vi "Process.vi"(8 "error in":errorcluster, 11 "Instrument.Example":refnum<class "Instrument.OxfordVRM.lvclass">) -> (0 "error out":errorcluster, 3 "Instrument.Example out":refnum<class "Instrument.OxfordVRM.lvclass">)   [LabVIEW 2016, in "Instrument.OxfordVRM.lvclass"]
doc: "---------------------------------------------------------------\nJKI State Machine Objects™\nhttp://jki.net/state-machine-objects/\nCopyright (C) 2005-2015, JKI <info@jki.net>\nALL RIGHTS RESERVED"
uses:
  Instrument.OxfordVRM.lvclass
  <vilib>/JKI/JKI SMO/SMO/SMO.lvclass
  <vilib>/JKI/JKI SMO/SMO/Typedefs/Parent Call--Enum.ctl
  <userlib>/LevyLab/Levylab Instruments/Instrument Types/Cryostat/Instrument.Cryostat.lvclass
  C:/Program Files (x86)/National Instruments/LabVIEW 2016/user.lib/LevyLab/Levylab Instruments/Instrument Types/Cryostat/Instrument.Cryostat.lvclass
  C:/Program Files (x86)/National Instruments/LabVIEW 2016/user.lib/LevyLab/Levylab Instruments/SMOs/Instrument/Instrument.lvclass
  C:/Program Files (x86)/National Instruments/LabVIEW 2016/vi.lib/JKI/JKI SMO/SMO/SMO.lvclass
  <userlib>/LevyLab/Levylab Instruments/Instrument Types/Cryostat/Typedefs/VRM Magnet Axis--Enum.ctl
panel:
  out "State":string
  out "timer":u32
  # "For instructions on how to use the JKI State Machine Objects, examples and video tutorials, visit:\nhttp://jki.net/state-machine-objects/\n\nJKI State Machine Objects™\nhttp://jki.net/state-machine-objects/\nCopyright (C) 2005-2015, JKI <info@jki.net>\nALL RIGHTS RESERVED"
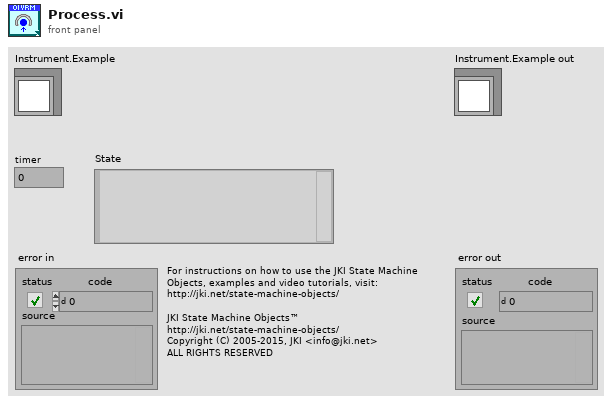
[diagram p1: front panel]
types:
  T1 = typedef "SMO.lvclass/Parent Call--Enum.ctl" = enum16{"Allows parent to run", "Does not request parent to run"}
  T2 = enum32{"invalid app kind", "Development System", "Run Time System", "Student Edition", "Embedded LabVIEW", "Evaluation", "Custom"}
  T3 = enum32{"Invalid", "Standard", "Closed", "Hidden", "Minimized", "Maximized"}
  T4 = enum32{"Bad", "Idle", "Run top level", "Running"}
  T5 = typedef "Instrument.OxfordVRM.lvclass/VRM Magnet Axis--Enum.ctl" = enum16{"Z", "X", "Y", "ALL"}
  T6 = cluster{"Core":cluster{"Current VI Reference":refnum<vi>, "Close Panel on Exit?":bool, "error":errorcluster}, "Self Reference":refnum<class "Instrument.OxfordVRM.lvclass">, "Field (T)":dbl, "Field Rate (T/min)":dbl, "Axis":T5, "Running Step":i32, "sequence":string[]}
  T7 = cluster{"Current VI Reference":refnum<vi>, "Close Panel on Exit?":bool, "error":errorcluster}
  T8 = typedef "SMO.lvclass/Protected Events.ctl" = cluster{"StopProcesses":refnum<user-event>, "AbortProcesses":refnum<user-event>, "Config Changed":refnum<user-event>, "Dependency":refnum<user-event>}
  T9 = typedef "Instrument.OxfordVRM.lvclass/PrivateEvents--Cluster.ctl" = cluster{"SequenceSetMagnetField":refnum<user-event>, "AbortSequence":refnum<user-event>}
  T10 = cluster{"Holding":bool, "Ramp to Setpoint":bool, "Ramp to Zero":bool, "Clamp":bool}
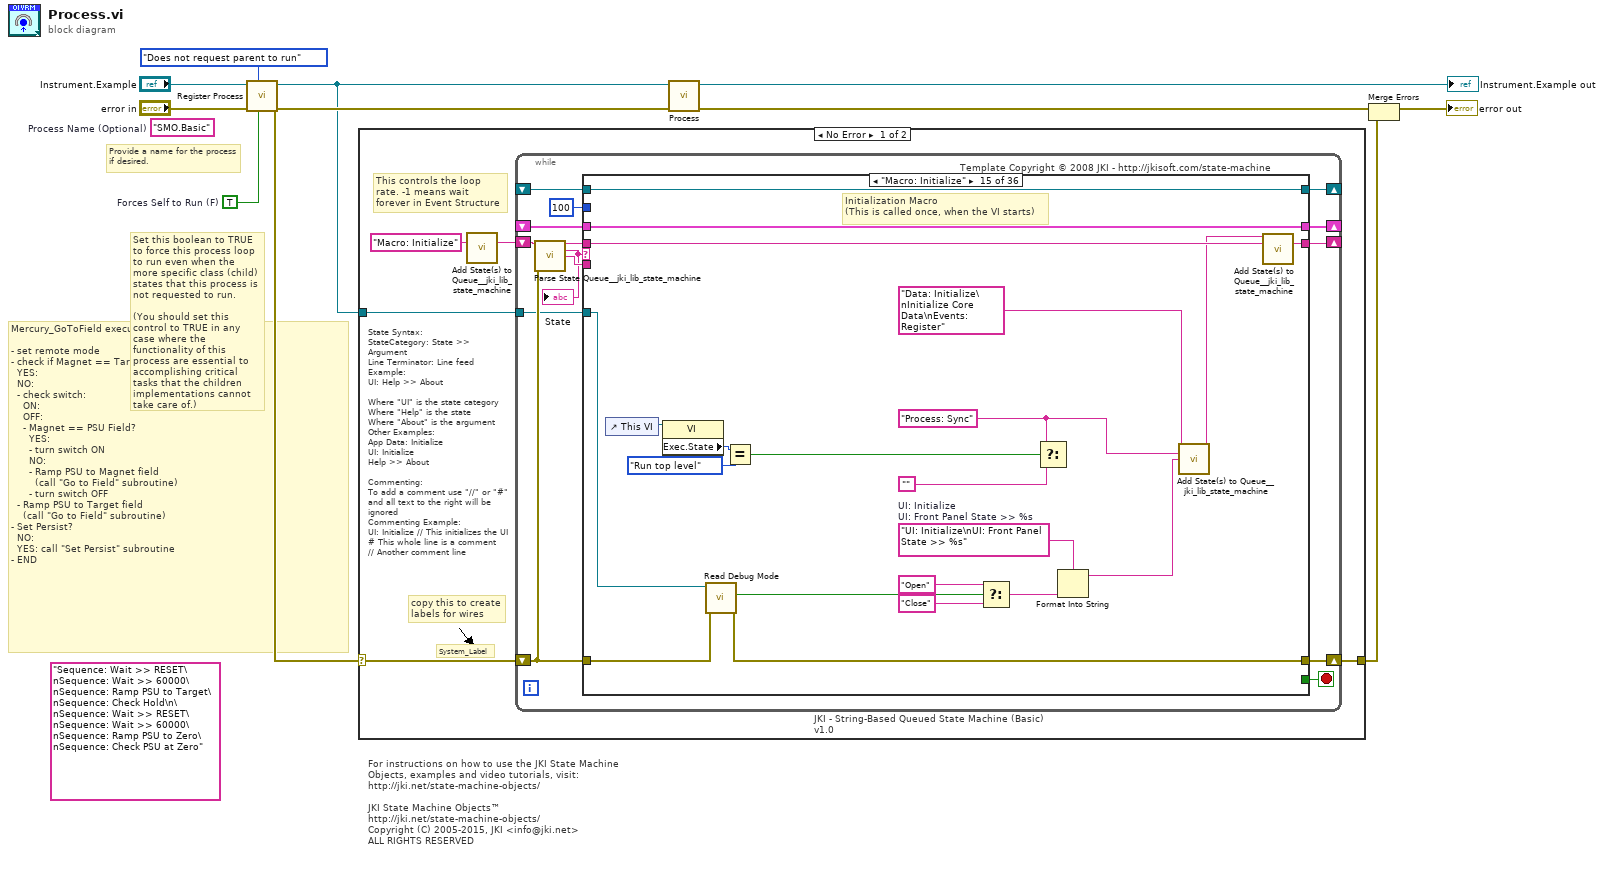
[diagram p0: block diagram]
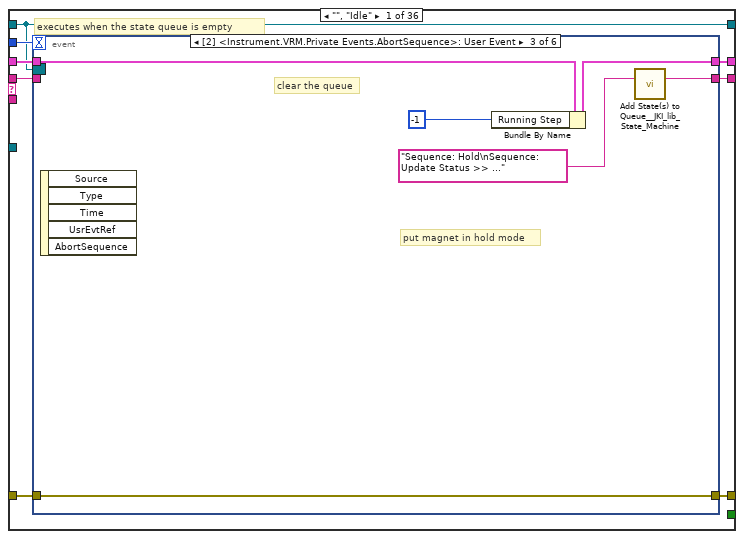
[diagram p2: hidden frame]
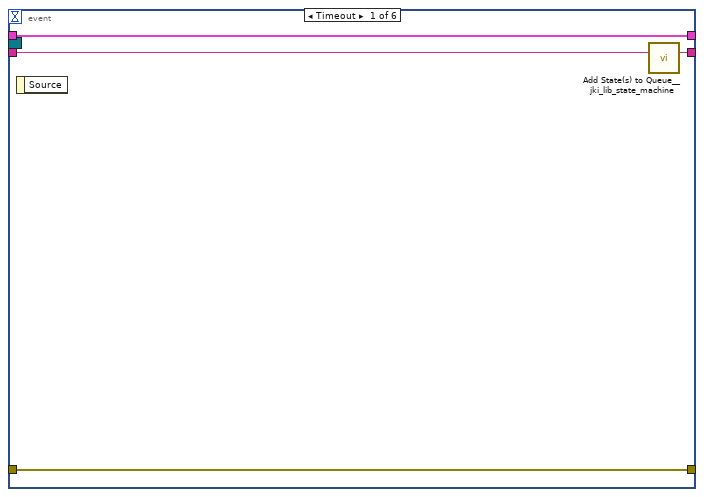
[diagram p3: hidden frame]
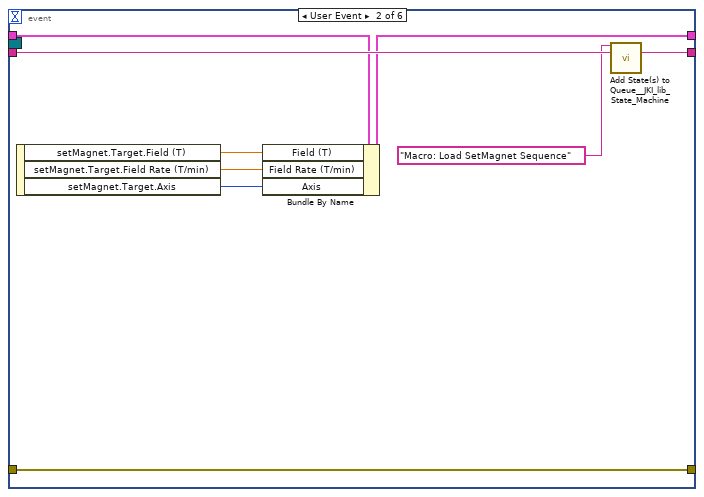
[diagram p4: hidden frame]
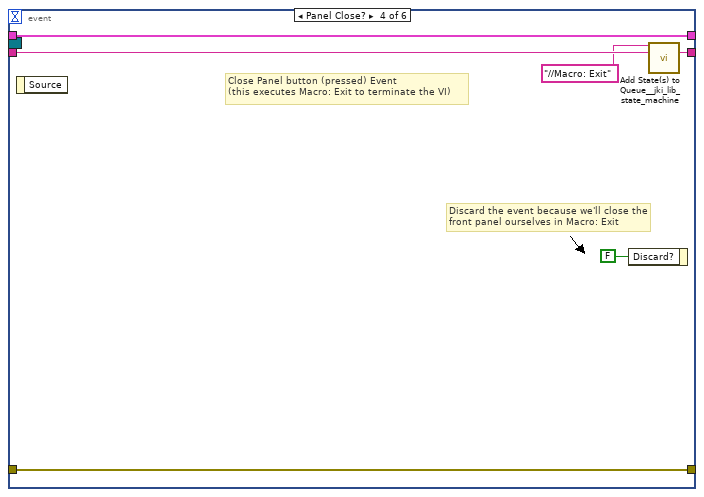
[diagram p5: hidden frame]
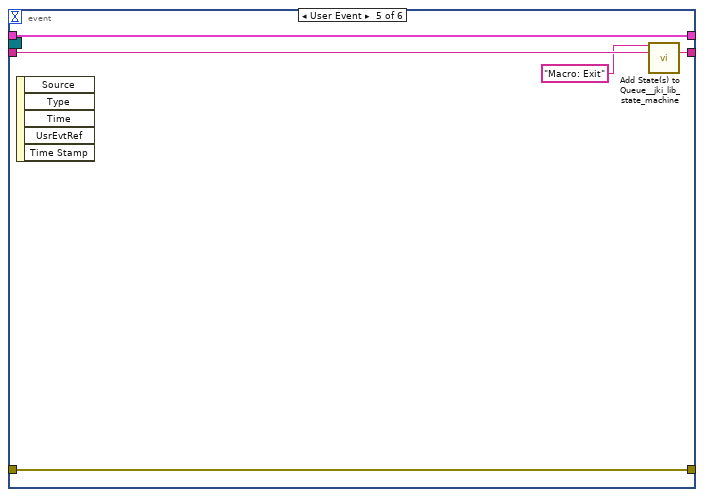
[diagram p6: hidden frame]
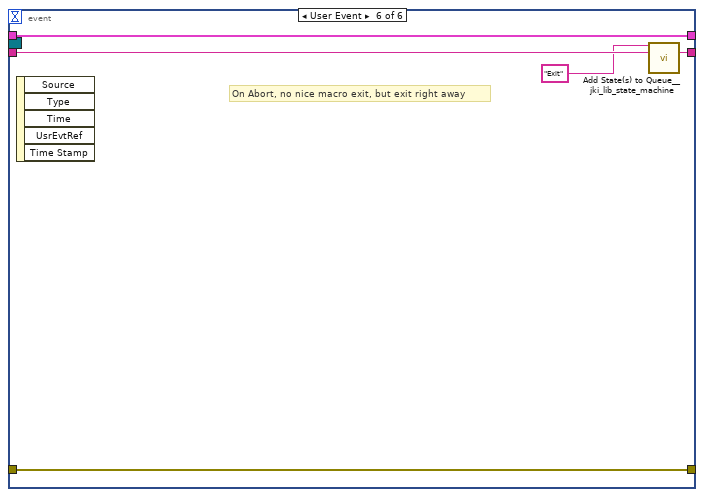
[diagram p7: hidden frame]
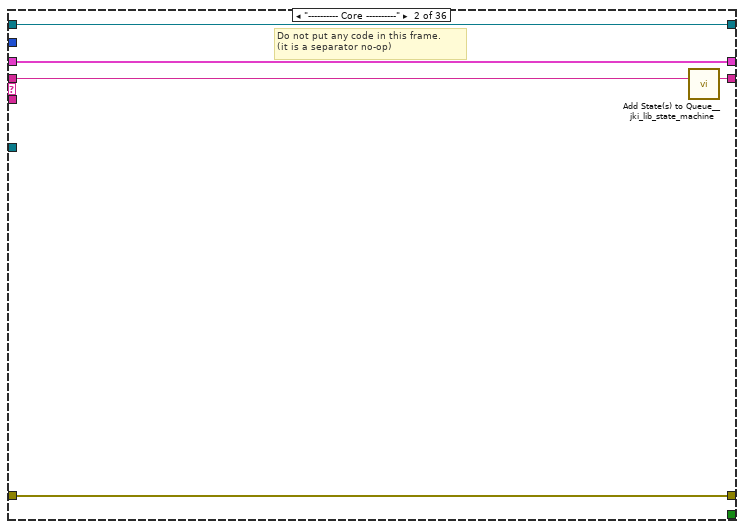
[diagram p8: hidden frame]
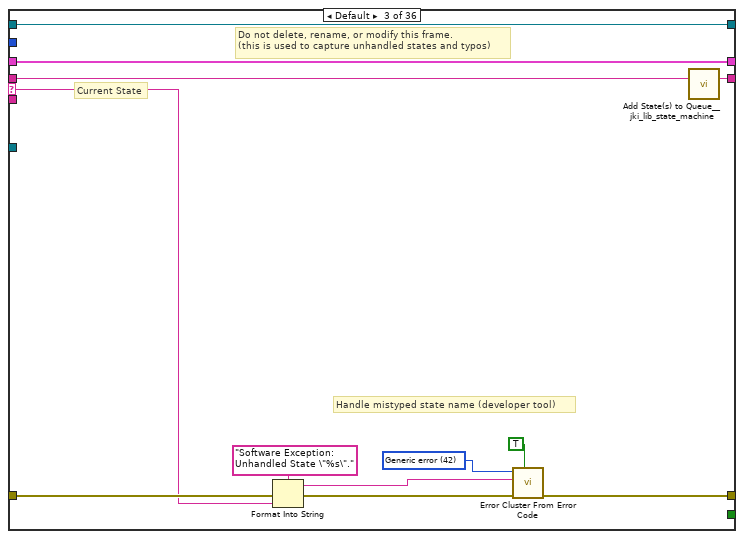
[diagram p9: hidden frame]
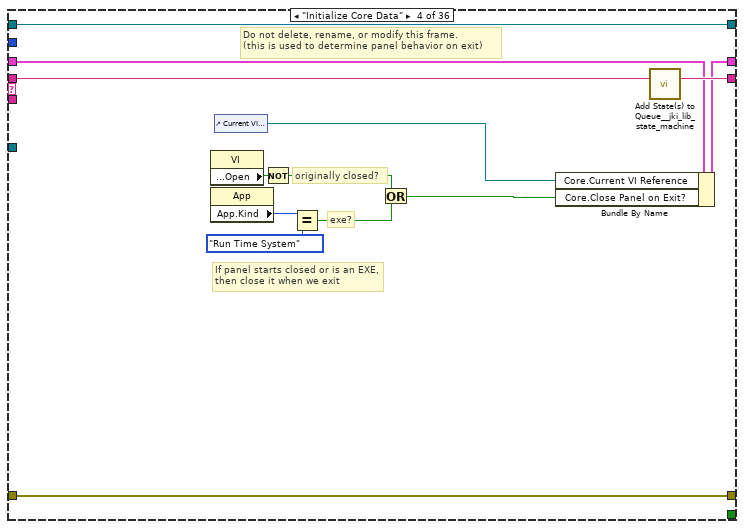
[diagram p10: hidden frame]
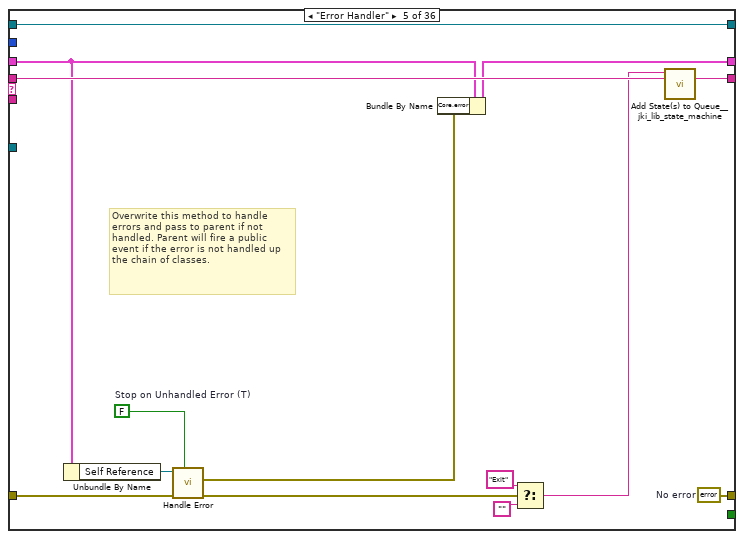
[diagram p11: hidden frame]
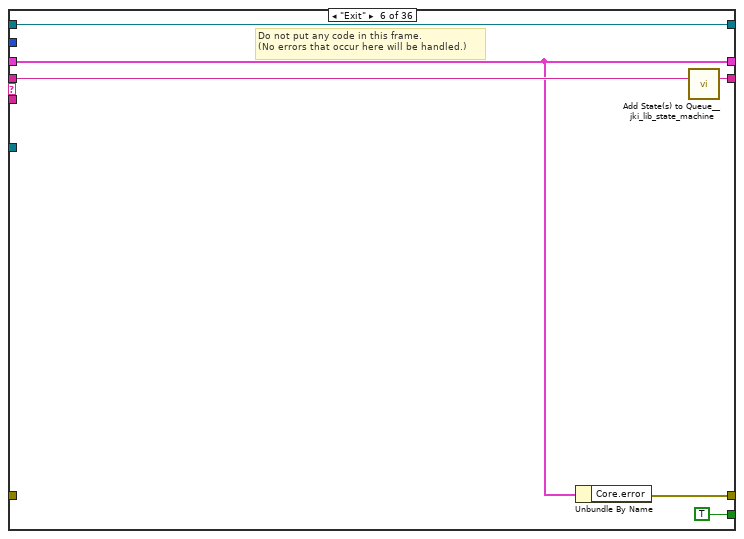
[diagram p12: hidden frame]
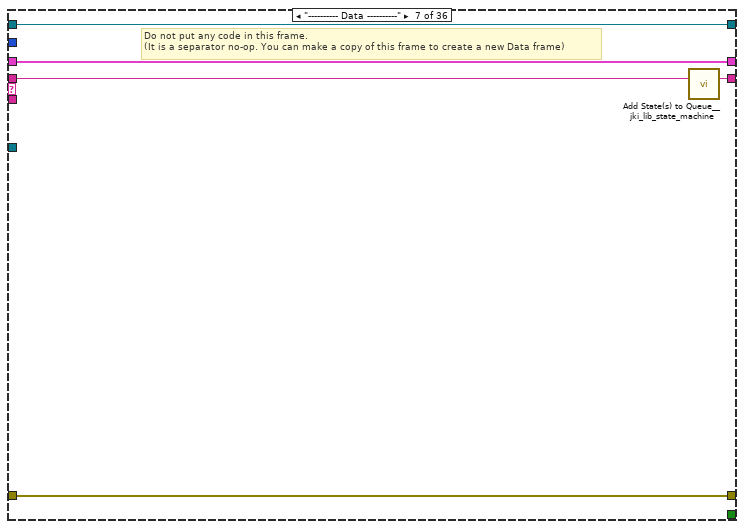
[diagram p13: hidden frame]
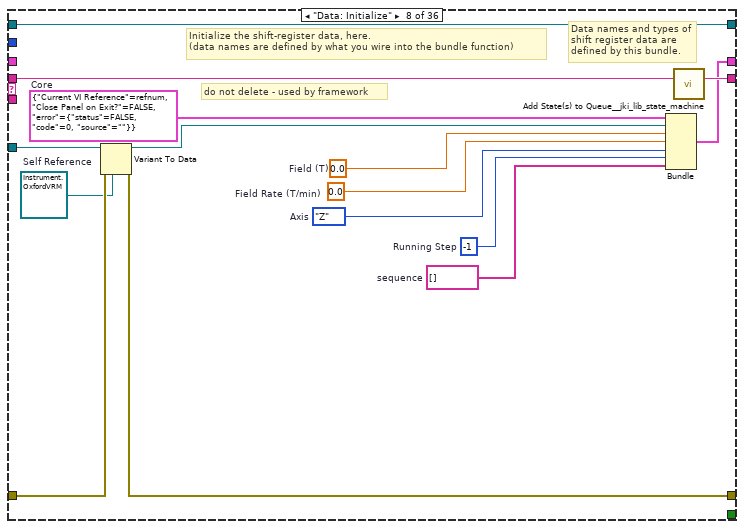
[diagram p14: hidden frame]
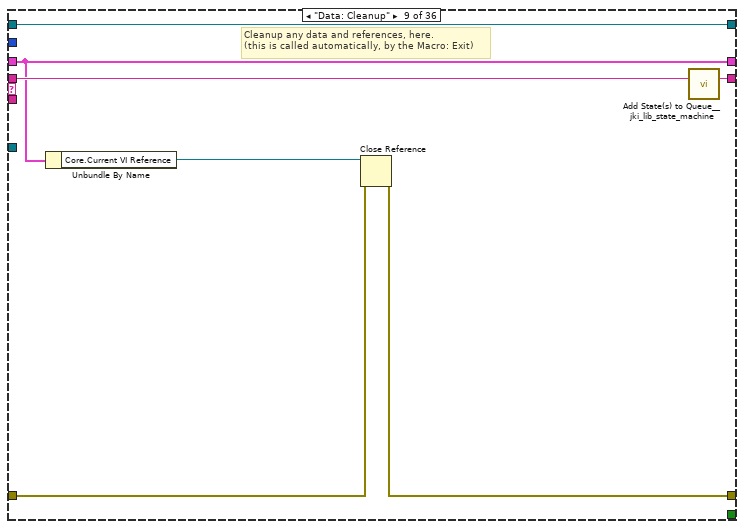
[diagram p15: hidden frame]
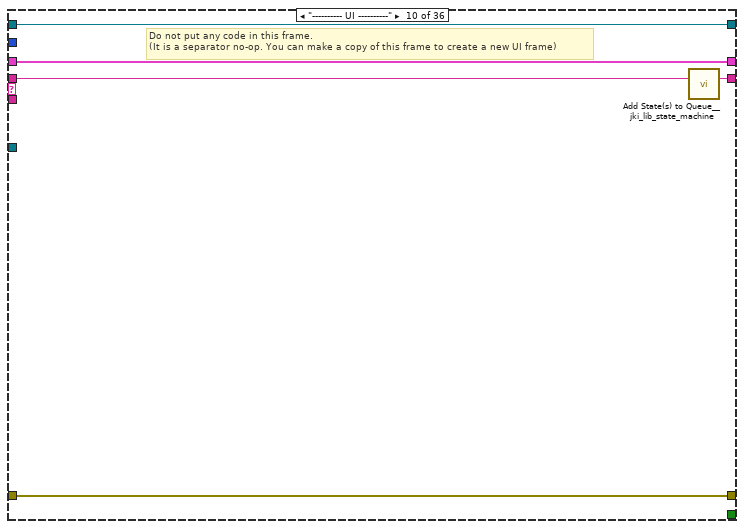
[diagram p16: hidden frame]
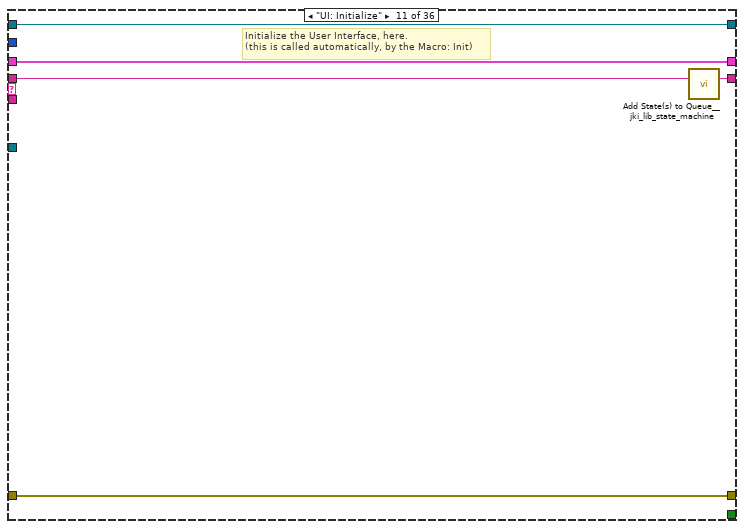
[diagram p17: hidden frame]
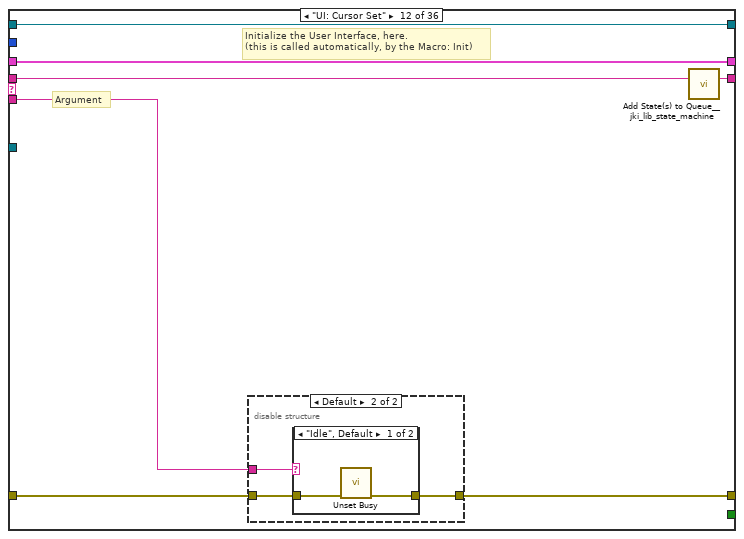
[diagram p18: hidden frame]
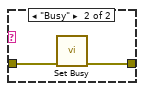
[diagram p20: hidden frame]
diagram:
  (unwired) "Sequence: Wait >> RESET\nSequence: Wait >> 60000\nSequence: Ramp PSU to Target\nSequence: Check Hold\n\nSequence: Wait >> RESET\nSequence: Wait >> 60000\nSequence: Ramp PSU to Zero\nSequence: Check PSU at Zero" ("State(s) in Front (\"\")")
  w1 = TRUE  # Forces Self to Run (F)
  (unwired) "SMO.Basic"  # Process Name (Optional)
  # "Mercury_GoToField executes the following states:\n\n- set remote mode\n- check if Magnet == Target.\n  YES:\n  NO:\n  - check switch:\n    ON:\n    OFF:\n    - Magnet == PSU Field?\n      YES:\n      - turn switch ON\n      NO:\n      - Ramp PSU to Magnet field\n        (call \"Go to Field\" subroutine)\n      - turn switch OFF\n  - Ramp PSU to Target field\n    (call \"Go to Field\" subroutine)\n- Set Persist?\n  NO:\n  YES: call \"Set Persist\" subroutine\n- END"
  # "Provide a name for the process\nif desired."
  # "Set this boolean to TRUE to force this process loop to run even when the more specific class (child) states that this process is not requested to run.\n\n(You should set this control to TRUE in any case where the functionality of this process are essential to accomplishing critical tasks that the children implementations cannot take care of.)"
  # "For instructions on how to use the JKI State Machine Objects, examples and video tutorials, visit:\nhttp://jki.net/state-machine-objects/\n\nJKI State Machine Objects™\nhttp://jki.net/state-machine-objects/\nCopyright (C) 2005-2015, JKI <info@jki.net>\nALL RIGHTS RESERVED"
  n1 = call <vilib>:"Register Process.vi"("Forces Self to Run (F)"=w1, "Parent Call"=Parent_Call--Enum."Does not request parent to run", "error in (no error)"="error in", "SMO"="Instrument.Example") -> ("error out"=w7:errorcluster, "SMO out"=w6:refnum<class "Instrument.OxfordVRM.lvclass">)  [unwired: 6 in]
  n2 = case shown="No Error" w7 {
    selector: w7 -> [w12 w596]
    tunnel: w6 -> [w13 _]
    tunnel: [w11 w596] -> w3
    frame No Error {
      # "State Syntax:\nStateCategory: State >> Argument\nLine Terminator: Line feed\nExample:\nUI: Help >> About\n\nWhere \"UI\" is the state category\nWhere \"Help\" is the state\nWhere \"About\" is the argument\nOther Examples:\nApp Data: Initialize\nUI: Initialize\nHelp >> About\n\nCommenting:\nTo add a comment use \"//\" or \"#\" and all text to the right will be ignored\nCommenting Example:\nUI: Initialize // This initializes the UI\n# This whole line is a comment\n// Another comment line"
      # "copy this to create labels for wires"
      # "This controls the loop rate. -1 means wait forever in Event Structure"
      # "System_Label"
      n3 = call <vilib>:"Add State(s) to Queue__jki_lib_state_machine.vi"("State(s) in (\"\")"="Macro: Initialize") -> ("States Out"=w15:string)  [unwired: 14 in]
      n4 = while "JKI - String-Based Queued State Machine (Basic) v1.0" {
        shift-right: [w23] -> _
        shift-left: _ -> [w22]
        shift-right: [w26] -> w11
        shift-left: w12 -> [w20]
        shift-right: [w25] -> _
        shift-left: w15 -> [w27]
        tunnel: w13 -> [w19]
        shift-right: [w18] -> _
        shift-left: _ -> [w17]
        stop <- w24 stop-if-true
        # "Template Copyright © 2008 JKI - http://jkisoft.com/state-machine"
        n5 = call <vilib>:"Parse State Queue__jki_lib_state_machine.vi"("State Queue"=w27, "Error In (no error)"=w20) -> ("Remaining States"=w29:string, "Current State"=w16:string, "Arguments"=w28:string)  [unwired: 11 in]
        "State" <- w16
        n6 = case shown="\"Macro: Initialize\"" w16 {
          selector: w16 -> [_ _ w79 _ _ _ _ _ _ _ _ _ _ _ _ _ _ _ _ _ _ _ _ _ _ _ w360 w385 w410 w441 w475 w494 w515 w536 w555 w586]
          tunnel: w29 -> [w37 w77 w83 w102 w116 w122 w127 w142 w149 w154 w159 w166 w182 w214 w235 w249 w266 _ w293 w304 w309 w322 w328 w337 w344 w354 w369 w398 w426 w458 w483 w504 w525 w546 w567 w595]
          tunnel: w28 -> [_ _ _ _ _ _ _ _ _ _ _ w160 w176 _ _ _ _ _ _ _ _ _ _ _ _ w346 _ w386 _ _ _ _ _ _ _ _]
          tunnel: w22 -> [w35 w74 w81 w93 w110 w118 w124 _ w144 w151 w157 w164 w178 w211 w232 w240 w254 w275 w290 w301 w306 w320 w326 w331 w340 w345 w366 w371 w419 w454 w480 w497 w518 w539 w564 w592]
          tunnel: [w34 w75 w85 w99 w111 w117 w125 w138 w145 w152 w156 w161 w179 w212 w215 w247 w264 w271 w291 w295 w307 w315 w324 w334 w341 w348 w363 w375 w413 w450 w471 w486 w507 w528 w547 w585] -> w26
          tunnel: w20 -> [w33 w75 w84 w99 w112 _ w125 w139 w146 w152 w156 w162 w180 w212 w216 w247 w264 w272 w291 w296 w307 w316 w324 w334 w341 w349 w358 w374 w408 w439 w472 w484 w506 w527 w549 w580]
          tunnel: [w36 w76 w82 w101 w115 w121 w126 w141 w148 w153 w158 w165 w181 w213 w234 w248 w265 w281 w292 w303 w308 w321 w327 w336 w343 w353 w368 w397 w425 w457 w482 w503 w524 w545 w566 w594] -> w25
          tunnel: [_ _ _ _ _ TRUE _ _ _ _ _ _ _ _ _ _ _ _ _ _ _ _ _ _ _ _ _ _ _ _ _ _ _ _ _ _] -> w24
          tunnel: [w32 w74 w81 w100 w109 w118 w124 w140 w144 w151 w157 w164 w178 w211 w232 w240 w262 w276 w290 w301 w306 w320 w326 w330 w339 w351 w365 w395 w418 w453 w479 w496 w517 w538 w563 w591] -> w23
          tunnel: 100 ("Timeout") -> [w31 _ _ _ _ _ _ _ _ _ _ _ _ _ _ _ _ _ _ _ _ _ _ _ _ _ _ _ _ _ _ _ _ _ _ _]
          tunnel: w19 -> [_ _ _ _ _ _ _ w136 _ _ _ _ _ _ w223 _ _ _ _ _ _ _ _ _ _ _ _ _ _ _ _ _ _ _ _ _]
          tunnel: [w30 w73 w78 w90 w114 w119 w123 w134 w143 w150 w155 w163 w175 w210 w233 w241 w263 w280 w289 w302 w305 w319 w325 w335 w342 w352 w367 w396 w424 w456 w481 w502 w523 w544 w565 w593] -> w18
          tunnel: w17 -> [w30 w73 w78 w90 w114 w119 w123 w134 w143 w150 w155 w163 w175 w210 w233 w241 w263 w280 w289 w302 w305 _ w325 w335 w342 w352 w367 w396 w424 w456 w481 w502 w523 w544 w565 w593]
          frame "", "Idle" {
            # "executes when the state queue is empty"
            n7 = event shown="[2] <Instrument.VRM.Private Events.AbortSequence>: User Event" {
              selector: w30 -> [_ _ _ _ _ _]
              dyn-events: _ -> [_ _ _ _ _ _]
              timeout: w31 -> [_ _ _ _ _ _]
              tunnel: w37 -> [w41 w48 _ w62 w67 w72]
              tunnel: [w40 w49 w55 w61 w66 w71] -> w36
              tunnel: w35 -> [w38 w45 w53 w59 w64 w69]
              tunnel: [w39 w50 w56 w60 w65 w70] -> w34
              tunnel: w33 -> [w39 w50 w56 w60 w65 w70]
              tunnel: [w38 w44 w52 w59 w64 w69] -> w32
              event Timeout {
                n8 = event-data() -> ()  [unwired: 1 in, 1 out]
                n9 = call <vilib>:"Add State(s) to Queue__jki_lib_state_machine.vi"("State(s) in (\"\")"=w41) -> ("States Out"=w40:string)  [unwired: 14 in]
              }
              event User Event {
                n10 = event-data() -> ("setMagnet.Target.Field (T)"=w47:dbl, "setMagnet.Target.Field Rate (T/min)"=w46:dbl, "setMagnet.Target.Axis"=w42:T5)  [unwired: 1 in]
                n11 = Bundle By Name(cluster=w45, "Field (T)"=w47, "Field Rate (T/min)"=w46, "Axis"=w42) -> (w44:T6)
                n12 = call <vilib>:"Add State(s) to Queue__JKI_lib_State_Machine.vi"("State(s) in Front (\"\")"="Macro: Load SetMagnet Sequence" ("State(s) at Back (\"\")"), "State(s) in (\"\")"=w48) -> ("States Out"=w49:string)  [unwired: 13 in]
              }
              event User Event {
                # "put magnet in hold mode"
                # "clear the queue"
                n13 = event-data() -> ()  [unwired: 1 in, 5 out]
                n14 = Bundle By Name(cluster=w53, "Running Step"=-1) -> (w52:T6)
                n15 = call <vilib>:"Add State(s) to Queue__JKI_lib_State_Machine.vi"("State(s) in (\"\")"="Sequence: Hold\nSequence: Update Status >> ..." ("State(s) at Back (\"\")")) -> ("States Out"=w55:string)  [unwired: 14 in]
              }
              event Panel Close? {
                # "Discard the event because we'll close the front panel ourselves in Macro: Exit"
                # "Close Panel button (pressed) Event\n(this executes Macro: Exit to terminate the VI)"
                n16 = event-data() -> ()  [unwired: 1 in, 1 out]
                n17 = event-data("Discard?"=FALSE) -> ()  [unwired: 1 in, 1 out]
                n18 = call <vilib>:"Add State(s) to Queue__jki_lib_state_machine.vi"("State(s) in Front (\"\")"="//Macro: Exit", "State(s) in (\"\")"=w62) -> ("States Out"=w61:string)  [unwired: 13 in]
              }
              event User Event {
                n19 = event-data() -> ()  [unwired: 1 in, 5 out]
                n20 = call <vilib>:"Add State(s) to Queue__jki_lib_state_machine.vi"("State(s) in Front (\"\")"="Macro: Exit", "State(s) in (\"\")"=w67) -> ("States Out"=w66:string)  [unwired: 13 in]
              }
              event User Event {
                # "On Abort, no nice macro exit, but exit right away"
                n21 = event-data() -> ()  [unwired: 1 in, 5 out]
                n22 = call <vilib>:"Add State(s) to Queue__jki_lib_state_machine.vi"("State(s) in Front (\"\")"="Exit", "State(s) in (\"\")"=w72) -> ("States Out"=w71:string)  [unwired: 13 in]
              }
            }
          }
          frame "---------- Core ----------" {
            # "Do not put any code in this frame.\n(it is a separator no-op)"
            n23 = call <vilib>:"Add State(s) to Queue__jki_lib_state_machine.vi"("State(s) in (\"\")"=w77) -> ("States Out"=w76:string)  [unwired: 14 in]
          }
          frame Default {
            w88 = 42 items=["No error", "Argument error", "Memory is full", "Out of zone", "End of file", "File already open", "Generic file I/O error", "File not found", "File permission error", "Disk is full", "Duplicate path", "Too many files open", "System feature not enabled", "Resource file not found", "Cannot add resource", "Resource not found", "Image not found", "Image memory error", "Pen does not exist", "Config type invalid", "Config token not found", "Config parse error", "Config memory error", "Bad external code format", "Bad external code offset", "External code not present", "Null window", "Destroy window error", "Null menu", "Print aborted", "Bad print record", "Print driver error", "Windows error during printing", "Memory error during printing", "Print dialog error", "Generic print error", "Invalid device refnum", "Device not found", "Device parameter error", "Device unit error", "Cannot open device", "Device call aborted", "Generic error", "Cancelled by user", "Object ID too low", "Object ID too high", "Object not in heap", "Unknown heap", "Unknown object (invalid DefProc)", "Unknown object (DefProc not in table)", "Message out of range", "Invalid (null) method", "Unknown message", "Manager call not supported", "Bad address", "Network operation in progress", "Network operation timed out", "Connection is busy", "Network attribute not supported", "Network error", "Address in use", "System out of memory", "Connection aborted", "Connection refused", "Not connected", "Already connected", "Connection closed", "Initialization error (interapplication manager)", "Bad occurrence", "Wait on unbound occurrence handler", "Occurrence queue overflow", "Datalog type conflict", "Unused", "Unrecognized type (interapplication manager)", "Memory corrupt", "Failed to make temporary DLL", "Old CIN version", "Drag socket not found", "Failed to load drop-object", "Failed to register OLE object", "Failed to release OLE object", "Format specifier type mismatch", "Unknown format specifier", "Too few format specifiers", "Too many format specifiers", "Scan failed", "Newer CIN version", "Error converting to variant", "Runtime menu error", "Password tampered", "Variant attribute not found", "Incompatible variant data type", "Event data is not available", "Event Store is not present", "Occurrence is not found", "Event Queue is not created", "Event info is not available", "Refnum passed is NULL", "Error retrieving Class GUID", "Error retrieving CoClass GUID", "Error retrieving TypeLib GUID.", "Bad built application magic bytes.", "Specific driver is different from the specific driver associated with the Logical Name.", "There is no session opened to the class driver.", "Max Error", "MAX - Error with config objects", "MAX - Error loading configuration", "MAX - Group not supported"]
            # "Current State"
            # "Do not delete, rename, or modify this frame.\n(this is used to capture unhandled states and typos)"
            # "Handle mistyped state name (developer tool)"
            n24 = Format Into String(format string="Software Exception: Unhandled State \"%s\"." ("message"), error in=w84, w79) -> (resulting string=w87:string, error out=w86:errorcluster)  [unwired: 1 in]
            n25 = call <vilib>:"Error Cluster From Error Code.vi"("show call chain? (False)"=TRUE, "error in (no error)"=w86, "error message (\"\")"=w87, "error code (0)"=w88) -> ("error out"=w85:errorcluster)  [unwired: 5 in]
            n26 = call <vilib>:"Add State(s) to Queue__jki_lib_state_machine.vi"("State(s) in (\"\")"=w83) -> ("States Out"=w82:string)  [unwired: 14 in]
          }
          frame "Initialize Core Data" {
            # "Do not delete, rename, or modify this frame.\n(this is used to determine panel behavior on exit)"
            # "originally closed?"
            # "exe?"
            # "If panel starts closed or is an EXE, then close it when we exit"
            n27 = property class="VI"() -> ("Front Panel.Open"=w98:bool)  [unwired: 2 in, 2 out]
            n28 = property class="App"() -> ("App.Kind"=w97:T2)  [unwired: 2 in, 2 out]
            n29 = control-ref of="Current VI Reference"() -> (w91:refnum<vi>)
            n30 = Not(x=w98) -> (.not. x?=w95:bool)
            n31 = Equal?(x=w97, y=T2."Run Time System" ("Application:Kind")) -> (x = y?=w94:bool)
            n32 = Or(x=w95, y=w94) -> (x .or. y?=w92:bool)
            n33 = Bundle By Name(cluster=w93, "Core.Current VI Reference"=w91, "Core.Close Panel on Exit?"=w92) -> (w100:T6)
            n34 = call <vilib>:"Add State(s) to Queue__jki_lib_state_machine.vi"("State(s) in (\"\")"=w102) -> ("States Out"=w101:string)  [unwired: 14 in]
          }
          frame "Error Handler" {
            w103 = FALSE  # Stop on Unhandled Error (T)
            w111 = errorcluster {"status"=FALSE, "code"=0, "source"=""}  # No error
            # "Overwrite this method to handle errors and pass to parent if not handled. Parent will fire a public event if the error is not handled up the chain of classes."
            n35 = Unbundle By Name(w110) -> ("Self Reference"=w113:refnum<class "Instrument.OxfordVRM.lvclass">)
            n36 = call-dynamic "Handle Error.vi"("Stop on Unhandled Error (T)"=w103, "error in"=w112, "Instrument"=w113) -> ("handling error"=w104:errorcluster, "Unhandled error"=w107:errorcluster)  [unwired: 6 in, 1 out]
            n37 = Bundle By Name(cluster=w110, "Core.error"=w107) -> (w109:T6)
            n38 = Select(t="Exit", s=w104, f="") -> (s? t:f=w108:string)
            n39 = call <vilib>:"Add State(s) to Queue__jki_lib_state_machine.vi"("State(s) in Front (\"\")"=w108, "State(s) in (\"\")"=w116) -> ("States Out"=w115:string)  [unwired: 13 in]
          }
          frame "Exit" {
            # "Do not put any code in this frame.\n(No errors that occur here will be handled.)"
            n40 = Unbundle By Name(w118) -> ("Core.error"=w117:errorcluster)
            n41 = call <vilib>:"Add State(s) to Queue__jki_lib_state_machine.vi"("State(s) in (\"\")"=w122) -> ("States Out"=w121:string)  [unwired: 14 in]
          }
          frame "---------- Data ----------" {
            # "Do not put any code in this frame.\n(It is a separator no-op. You can make a copy of this frame to create a new Data frame)"
            n42 = call <vilib>:"Add State(s) to Queue__jki_lib_state_machine.vi"("State(s) in (\"\")"=w127) -> ("States Out"=w126:string)  [unwired: 14 in]
          }
          frame "Data: Initialize" {
            w128 = VRM_Magnet_Axis--Enum."Z"  # Axis
            w129 = string[] []  # sequence
            w130 = -1  # Running Step
            w131 = 0.0  # Field Rate (T/min)
            w132 = 0.0  # Field (T)
            w133 = T7 {"Current VI Reference"=refnum, "Close Panel on Exit?"=FALSE, "error"={"status"=FALSE, "code"=0, "source"=""}}  # Core
            w137 = refnum<class "Instrument.OxfordVRM.lvclass"> refnum  # Self Reference
            # "do not delete - used by framework"
            # "Data names and types of shift register data are defined by this bundle."
            # "Initialize the shift-register data, here.\n(data names are defined by what you wire into the bundle function)"
            n43 = Variant To Data(error in=w139, type=w137, Variant=w136) -> (data=w135:refnum<class "Instrument.OxfordVRM.lvclass">, error out=w138:errorcluster)
            n44 = Bundle("Core"=w133, "Self Reference"=w135, "Field (T)"=w132, "Field Rate (T/min)"=w131, "Axis"=w128, "Running Step"=w130, "sequence"=w129) -> (w140:T6)  [unwired: 1 in]
            n45 = call <vilib>:"Add State(s) to Queue__jki_lib_state_machine.vi"("State(s) in (\"\")"=w142) -> ("States Out"=w141:string)  [unwired: 14 in]
          }
          frame "Data: Cleanup" {
            # "Cleanup any data and references, here.\n(this is called automatically, by the Macro: Exit)"
            n46 = Unbundle By Name(w144) -> ("Core.Current VI Reference"=w147:refnum<vi>)
            n47 = Close Reference(reference=w147, error in (no error)=w146) -> (error out=w145:errorcluster)
            n48 = call <vilib>:"Add State(s) to Queue__jki_lib_state_machine.vi"("State(s) in (\"\")"=w149) -> ("States Out"=w148:string)  [unwired: 14 in]
          }
          frame "---------- UI ----------" {
            # "Do not put any code in this frame.\n(It is a separator no-op. You can make a copy of this frame to create a new UI frame)"
            n49 = call <vilib>:"Add State(s) to Queue__jki_lib_state_machine.vi"("State(s) in (\"\")"=w154) -> ("States Out"=w153:string)  [unwired: 14 in]
          }
          frame "UI: Initialize" {
            # "Initialize the User Interface, here.\n(this is called automatically, by the Macro: Init)"
            n50 = call <vilib>:"Add State(s) to Queue__jki_lib_state_machine.vi"("State(s) in (\"\")"=w159) -> ("States Out"=w158:string)  [unwired: 14 in]
          }
          frame "UI: Cursor Set" {
            # "Argument"
            # "Initialize the User Interface, here.\n(this is called automatically, by the Macro: Init)"
            n51 = disable-structure shown="Default" {
              disable-tunnel: w162 -> [w167 w170]
              disable-tunnel: [w167 w169] -> w161
              disable-tunnel: w160 -> [_ w168]
              frame condition #0 {
              }
              frame condition #1 (active) {
                n52 = case shown="\"Idle\", Default" w168 {
                  tunnel: w170 -> [w172 w174]
                  tunnel: [w171 w173] -> w169
                  frame "Idle", Default {
                    n53 = call <vilib>:"Unset Busy.vi"("error in (no error)"=w172) -> ("error out"=w171:errorcluster)  [unwired: 10 in]
                  }
                  frame "Busy" {
                    n54 = call <vilib>:"Set Busy.vi"("error in (no error)"=w174) -> ("error out"=w173:errorcluster)  [unwired: 9 in, 1 out]
                  }
                }
              }
            }
            n55 = call <vilib>:"Add State(s) to Queue__jki_lib_state_machine.vi"("State(s) in (\"\")"=w166) -> ("States Out"=w165:string)  [unwired: 14 in]
          }
          frame "UI: Front Panel State" {
            # "Argument"
            # "Set Front Panel Open or Closed\n(Usage: \"UI: Front Panel State >> Open|Close\")"
            n56 = Unbundle By Name(w178) -> ("Core.Current VI Reference"=w177:refnum<vi>)
            n57 = disable-structure shown="Default" {
              disable-tunnel: w180 -> [w186 w209]
              disable-tunnel: [w185 w209] -> w179
              disable-tunnel: w177 -> [w184 _]
              disable-tunnel: w176 -> [w183 _]
              frame condition #0 (active) {
                n58 = case shown="\"Close\"" w183 {
                  tunnel: w186 -> [w190 w203]
                  tunnel: [w192 w204] -> w185
                  tunnel: w184 -> [w191 w201]
                  frame "Open", Default {
                    n59 = property class="VI"(reference=w191, error in=w190) -> (reference out=w188:refnum<vi>, error out=w189:errorcluster, "FP.State"=w187:T3)
                    n60 = case shown="\"Closed\"" w187 {
                      tunnel: [w195 w198] -> w192
                      tunnel: w189 -> [w194 w198]
                      tunnel: w188 -> [w193 _]
                      frame "Closed" {
                        n61 = invoke class="VI" method="FP.Open"(reference=w193, error in=w194, "Activate"=TRUE, "State"=T3."Standard") -> (error out=w195:errorcluster)  [unwired: 1 in, 4 out]
                      }
                      frame Default {
                      }
                    }
                  }
                  frame "Close" {
                    n62 = property class="VI"(reference=w201, error in=w203) -> (reference out=w200:refnum<vi>, error out=w202:errorcluster, "FP.State"=w199:T3)
                    n63 = case shown="Default" w199 {
                      tunnel: [w205 w208] -> w204
                      tunnel: w202 -> [w205 w207]
                      tunnel: w200 -> [_ w206]
                      frame "Invalid", "Closed" {
                      }
                      frame Default {
                        n64 = invoke class="VI" method="FP.Close"(reference=w206, error in=w207) -> (error out=w208:errorcluster)  [unwired: 1 in, 2 out]
                      }
                    }
                  }
                }
              }
              frame condition #1 {
              }
            }
            n65 = call <vilib>:"Add State(s) to Queue__jki_lib_state_machine.vi"("State(s) in (\"\")"=w182) -> ("States Out"=w181:string)  [unwired: 14 in]
          }
          frame "---------- Macro ----------" {
            # "Do not put any code in this frame.\n(It is a separator no-op. You can make a copy of this frame to create a new Macro frame)"
            n66 = call <vilib>:"Add State(s) to Queue__jki_lib_state_machine.vi"("State(s) in (\"\")"=w214) -> ("States Out"=w213:string)  [unwired: 14 in]
          }
          frame "Macro: Initialize" {
            w218 = "UI: Initialize\nUI: Front Panel State >> %s"  # UI: Initialize UI: Front Panel State >> %s
            w224 = "Process: Sync"
            # "Initialization Macro\n(This is called once, when the VI starts)"
            n67 = control-ref of="This VI"() -> (w226:refnum<vi>)
            n68 = property class="VI"(reference=w226) -> ("Exec.State"=w225:T4)  [unwired: 1 in, 2 out]
            n69 = call-dynamic "Read Debug Mode.vi"("error in (no error)"=w216, "Instrument in"=w223) -> ("error out"=w215:errorcluster, "Debug Mode?"=w220:bool)  [unwired: 7 in, 1 out]
            n70 = Equal?(x=w225, y=T4."Run top level") -> (x = y?=w230:bool)
            n71 = Select(t="Open", s=w220, f="Close") -> (s? t:f=w219:string)
            n72 = Select(t=w224, s=w230, f="") -> ()  [unwired: 1 out]
            n73 = Format Into String(format string=w218, w219) -> (resulting string=w217:string)  [unwired: 2 in, 1 out]
            n74 = call <vilib>:"Add State(s) to Queue__jki_lib_state_machine.vi"("State(s) in Front (\"\")"="Data: Initialize\nInitialize Core Data\nEvents: Register", "State(s) in (\"\")"=w224, "State(s) at Back (\"\")"=w217) -> ("States Out"=w227:string)  [unwired: 12 in]
            n75 = call <vilib>:"Add State(s) to Queue__jki_lib_state_machine.vi"("State(s) in Front (\"\")"=w227, "State(s) in (\"\")"=w235) -> ("States Out"=w234:string)  [unwired: 13 in]
          }
          frame "Macro: Exit" {
            # "Exit Macro\n(This is called once, when the VI exits)"
            n76 = Unbundle By Name(w240) -> ("Core.Close Panel on Exit?"=w246:bool)
            n77 = Select(t="UI: Front Panel State >> Close", s=w246, f="") -> (s? t:f=w243:string)
            n78 = call <vilib>:"Add State(s) to Queue__jki_lib_state_machine.vi"("State(s) in Front (\"\")"="Data: Cleanup\nEvents: Unregister", "State(s) in (\"\")"="Process: Sync", "State(s) at Back (\"\")"="Exit") -> ("States Out"=w237:string)  [unwired: 12 in]
            n79 = call <vilib>:"Add State(s) to Queue__jki_lib_state_machine.vi"("State(s) in (\"\")"=w243, "State(s) at Back (\"\")"=w237) -> ("States Out"=w242:string)  [unwired: 13 in]
            n80 = call <vilib>:"Add State(s) to Queue__jki_lib_state_machine.vi"("State(s) in Front (\"\")"=w242, "State(s) in (\"\")"=w249) -> ("States Out"=w248:string)  [unwired: 13 in]
          }
          frame "Macro: Run Sequence" {
            # "0,1,2,3,4,"
            # "5"
            # "Do not put any code in this frame.\n(It is a separator no-op. You can make a copy of this frame to create a new Macro frame)"
            n81 = Unbundle By Name(w254) -> ("sequence"=w260:string[], "Running Step"=w252:i32)
            n82 = Index Array(array=w260, index=w252) -> (element=w258:string)
            n83 = Array Size(array=w260) -> (size(s)=w261:i32)
            n84 = Equal?(x=w261, y=w252) -> (x = y?=w253:bool)
            n85 = Select(t=-1 ("Running Step"), s=w253, f=w252) -> (s? t:f=w259:i32)
            n86 = Select(t="Sequence: Update Status >> ...", s=w253, f="Idle\nMacro: Run Sequence" ("State(s) at Back (\"\")")) -> (s? t:f=w255:string)
            n87 = Bundle By Name(cluster=w254, "Running Step"=w259) -> (w262:T6)
            n88 = call <vilib>:"Add State(s) to Queue__jki_lib_state_machine.vi"("State(s) in Front (\"\")"=w258, "State(s) at Back (\"\")"=w255) -> ("States Out"=w257:string)  [unwired: 13 in]
            n89 = call <vilib>:"Add State(s) to Queue__jki_lib_state_machine.vi"("State(s) in Front (\"\")"=w257, "State(s) in (\"\")"=w266) -> ("States Out"=w265:string)  [unwired: 13 in]
          }
          frame "Macro: Load SetMagnet Sequence" {
            # "clear the queue"
            # "Do not put any code in this frame.\n(It is a separator no-op. You can make a copy of this frame to create a new Macro frame)"
            n90 = Unbundle By Name(w275) -> ("Self Reference"=w274:refnum<class "Instrument.OxfordVRM.lvclass">, "Field (T)"=w270:dbl, "Axis"=w267:T5)
            n91 = call "Get Field.vi"("Axis"=w267, "error in (no error)"=w272, "Instrument.VRM in"=w274) -> ("error out"=w271:errorcluster, "Field (T)"=w269:dbl)  [unwired: 6 in, 1 out]
            n92 = call "FloatApprox.vi"("y"=w270, "x"=w269) -> ("x ~ y?"=w273:bool)  [unwired: 4 in]
            n93 = call <userlib>:"String to 1D Array__ogtk.vi"("delimiter (Tab)"="\n", "string"="Sequence: Hold\nSequence: Check Hold\nSequence: Ramp PSU to Target\nSequence: Check Hold" ("State(s) in Front (\"\")")) -> ("Array of Strings"=w279:string[])  [unwired: 9 in]
            n94 = case shown="False" w273 {
              tunnel: w279 -> [w285 _]
              tunnel: ["Macro: Run Sequence" ("State(s) in Front (\"\")") "" ("State(s) in Front (\"\")")] -> w278
              tunnel: [w283 w287] -> w276
              tunnel: w275 -> [w282 w287]
              frame False {
                n95 = Bundle By Name(cluster=w282, "Running Step"=0 ("sequence"), "sequence"=w285) -> (w283:T6)
              }
              frame True {
              }
            }
            n96 = call <vilib>:"Add State(s) to Queue__jki_lib_state_machine.vi"("State(s) in Front (\"\")"=w278) -> ("States Out"=w281:string)  [unwired: 14 in]
          }
          frame "---------- Process ----------" {
            # "Template Separator\n(You can make a copy of, or modify, this frame)"
            n97 = call <vilib>:"Add State(s) to Queue__jki_lib_state_machine.vi"("State(s) in (\"\")"=w293) -> ("States Out"=w292:string)  [unwired: 14 in]
          }
          frame "Process: Sync" {
            n98 = Unbundle By Name(w301) -> ("Self Reference"=w297:refnum<class "Instrument.OxfordVRM.lvclass">)
            n99 = call <vilib>:"WaitOnProcessSync.vi"("error in (no error)"=w296, "SMO"=w297) -> ("error out"=w295:errorcluster, "Don't run?"=w300:bool)  [unwired: 7 in, 1 out]
            n100 = Select(t="Data: Cleanup\nEvents: Unregister\nExit", s=w300, f="") -> (s? t:f=w294:string)
            n101 = call <vilib>:"Add State(s) to Queue__jki_lib_state_machine.vi"("State(s) in Front (\"\")"=w294, "State(s) in (\"\")"=w304) -> ("States Out"=w303:string)  [unwired: 13 in]
          }
          frame "---------- Events ----------" {
            # "Template Separator\n(You can make a copy of, or modify, this frame)"
            n102 = call <vilib>:"Add State(s) to Queue__jki_lib_state_machine.vi"("State(s) in (\"\")"=w309) -> ("States Out"=w308:string)  [unwired: 14 in]
          }
          frame "Events: Register" {
            # "Expand to add\nmore events"
            n103 = Unbundle By Name(w320) -> ("Self Reference"=w317:refnum<class "Instrument.OxfordVRM.lvclass">)
            n104 = call <vilib>:"GetProtectedEvents.vi"("SMO"=w317) -> ("error out"=w313:errorcluster, "SMO Protected Events"=w318:T8, "SMO out"=w312:refnum<class "Instrument.OxfordVRM.lvclass">)  [unwired: 8 in]
            n105 = call "Instrument.Oxford1820.GetPrivateEvents.vi"("Instrument.Oxford1820"=w312) -> ("error out"=w311:errorcluster, "Instrument.VRM.Private Events"=w310:T9)  [unwired: 8 in, 1 out]
            n106 = register-events(w318, w310) -> (reference out=w319:refnum<event-registration>, error out=w314:errorcluster)  [unwired: 2 in]
            n107 = Merge Errors(w311, w316, w314, w313) -> (w315:errorcluster)
            n108 = call <vilib>:"Add State(s) to Queue__jki_lib_state_machine.vi"("State(s) in (\"\")"=w322) -> ("States Out"=w321:string)  [unwired: 14 in]
          }
          frame "Events: Unregister" {
            n109 = Unregister For Events(event registration refnum=w325, error in=w324) -> (error out=w323:errorcluster)
            n110 = call <vilib>:"Clear Errors.vi"("error in (no error)"=w323) -> ()  [unwired: 5 in, 2 out]
            n111 = call <vilib>:"Add State(s) to Queue__jki_lib_state_machine.vi"("State(s) in (\"\")"=w328) -> ("States Out"=w327:string)  [unwired: 14 in]
          }
          frame "---------- Sequence ----------" {
            n112 = Unbundle By Name(w331) -> ("Running Step"=w329:i32, "Self Reference"=w333:refnum<class "Instrument.OxfordVRM.lvclass">)
            n113 = Increment(x=w329) -> (x+1=w332:i32)
            n114 = Bundle By Name(cluster=w331, "Running Step"=w332, "Self Reference"=w333) -> (w330:T6)
            n115 = call <vilib>:"Add State(s) to Queue__jki_lib_state_machine.vi"("State(s) in (\"\")"=w337) -> ("States Out"=w336:string)  [unwired: 14 in]
          }
          frame "Sequence: Template" {
            # "switch ON/OFF:\n- include checks for PSU == Magnet.\n- call \"Go to Field\" as needed to make PSU == Magnet"
            # "\"Set Persist\" subroutine:\n\n- switch on?\n  NO:\n  YES:\n  - turn switch OFF\n- Ramp PSU to 0\n  (call \"Go to Field\" subroutine)\n- END"
            # "\"Go to Field\" subroutine:\n\n- set to remote mode (obsolete?)\n- write target field.\n  check and resend if necessary\n- put in hold mode.\n  check and resend if necessary\n- check if Target = PSU:\n  YES:\n  NO:\n  - put in GTOS mode. check and resend if necessary\n- wait until PSU is in hold mode\n  (PSU will go to hold mode once PSU @ target)\n- END"
            # "Mercury_GoToField executes the following states:\n\n- set remote mode (obsolete?)\n- check if Magnet == Target.\n  YES:\n  NO:\n  - check switch:\n    ON:\n    OFF:\n    - Magnet == PSU Field?\n      YES:\n      - turn switch ON\n      NO:\n      - Ramp PSU to Magnet field\n        (call \"Go to Field\" subroutine)\n      - turn switch OFF\n  - Ramp PSU to Target field\n    (call \"Go to Field\" subroutine)\n- Set Persist?\n  NO:\n  YES: call \"Set Persist\" subroutine\n- END"
            n116 = Unbundle By Name(w340) -> ("Self Reference"=w338:refnum<class "Instrument.OxfordVRM.lvclass">)
            n117 = Bundle By Name(cluster=w340, "Self Reference"=w338) -> (w339:T6)
            n118 = call <vilib>:"Add State(s) to Queue__jki_lib_state_machine.vi"("State(s) in (\"\")"=w344) -> ("States Out"=w343:string)  [unwired: 14 in]
          }
          frame "Sequence: Update Status" {
            n119 = Unbundle By Name(w345) -> ("Self Reference"=w350:refnum<class "Instrument.OxfordVRM.lvclass">)
            n120 = call "Instrument.Oxford1820.ProcessStatus.vi"("error in (no error)"=w349, "event data"=w346, "Instrument.Oxford1820"=w350) -> ("error out"=w348:errorcluster, "Instrument.Oxford1820 out"=w347:refnum<class "Instrument.OxfordVRM.lvclass">)  [unwired: 7 in]
            n121 = Bundle By Name(cluster=w345, "Self Reference"=w347) -> (w351:T6)
            n122 = call <vilib>:"Add State(s) to Queue__jki_lib_state_machine.vi"("State(s) in (\"\")"=w354) -> ("States Out"=w353:string)  [unwired: 14 in]
          }
          frame "Sequence: Hold" {
            n123 = Unbundle By Name(w366) -> ("Running Step"=w357:i32, "Self Reference"=w359:refnum<class "Instrument.OxfordVRM.lvclass">, "Axis"=w355:T5)
            n124 = Increment(x=w357) -> (x+1=w356:i32)
            n125 = call "Hold.vi"("Axis"=w355, "error in (no error)"=w358, "Instrument.VRM in"=w359) -> ("error out"=w363:errorcluster, "Instrument.VRM out"=w364:refnum<class "Instrument.OxfordVRM.lvclass">)  [unwired: 6 in, 1 out]
            n126 = Bundle By Name(cluster=w366, "Running Step"=w356, "Self Reference"=w364) -> (w365:T6)
            n127 = call <vilib>:"Build State String with Arguments__JKI_lib_State_Machine.vi"("Arguments (\"\")"=w360, "State"="Sequence: Update Status") -> ("State with Arguments"=w362:string)  [unwired: 4 in]
            n128 = call <vilib>:"Add State(s) to Queue__jki_lib_state_machine.vi"("State(s) in Front (\"\")"=w362, "State(s) in (\"\")"=w369) -> ("States Out"=w368:string)  [unwired: 13 in]
          }
          frame "Sequence: Wait" {
            # "F = repeat this state. wait\nT = go to next state. don't wait"
            n129 = Unbundle By Name(w371) -> ("Running Step"=w394:i32)
            n130 = Equal?(x=w386, y="RESET") -> (x = y?=w390:bool)
            n131 = case shown="False" w390 {
              tunnel: [w400 u32 10000 ("time (ms)")] -> w389
              tunnel: [w403 w405] -> w376
              tunnel: w374 -> [w402 w405]
              tunnel: w386 -> [w401 _]
              frame False {
                n132 = Scan From String(format string="%d", input string=w401, error in=w402) -> (error out=w403:errorcluster, output 1=w399:i32)  [unwired: 2 in, 2 out]
                n133 = To Unsigned Long Integer(number=w399) -> (unsigned 32bit integer=w400:u32)
              }
              frame True {
              }
            }
            n134 = call <userlib>:"Periodic Trigger__ogtk.vi"("time (ms)"=w389, "reset"=w390) -> ("Triggered"=w391:bool, "timer value"=w388:u32)  [unwired: 11 in, 1 out]
            n135 = Or(x=w391, y=w390) -> (x .or. y?=w373:bool)
            n136 = Increment(x=w394) -> (x+1=w393:i32)
            n137 = Subtract(x=w389, y=w388) -> (x-y=w380:u32)
            "timer" <- w380
            n138 = Select(t=u32 0, s=w373, f=u32 100 ("milliseconds to wait")) -> (s? t:f=w378:u32)
            n139 = Select(t=w393, s=w373, f=w394) -> (s? t:f=w392:i32)
            n140 = call <userlib>:"Wait (ms)__ogtk.vi"("error in (no error)"=w376, "milliseconds to wait"=w378) -> ("error out"=w375:errorcluster)  [unwired: 8 in, 1 out]
            n141 = Bundle By Name(cluster=w371, "Running Step"=w392) -> (w395:T6)
            n142 = Divide(x=w380, y=u32 1000) -> (x/y=w382:dbl)
            n143 = Format Into String(format string="%s >> %d s", w385, w382) -> (resulting string=w383:string)  [unwired: 2 in, 1 out]
            n144 = call <vilib>:"Build State String with Arguments__JKI_lib_State_Machine.vi"("Arguments (\"\")"=w383, "State"="Sequence: Update Status") -> ("State with Arguments"=w370:string)  [unwired: 4 in]
            n145 = call <vilib>:"Add State(s) to Queue__jki_lib_state_machine.vi"("State(s) in Front (\"\")"=w370, "State(s) in (\"\")"=w398) -> ("States Out"=w397:string)  [unwired: 13 in]
          }
          frame "Sequence: Ramp PSU to Target" {
            # "#todo: add abort public method"
            # "#todo: make these separate states\n1. check B = Target?\n2. Turn on switch\n3. set PSU to target\n4. check hold OR psu = target\n5. set persist mode"
            n146 = Unbundle By Name(w419) -> ("Running Step"=w417:i32, "Self Reference"=w409:refnum<class "Instrument.OxfordVRM.lvclass">, "Field (T)"=w414:dbl, "Field Rate (T/min)"=w415:dbl, "Axis"=w407:T5)
            n147 = Increment(x=w417) -> (x+1=w416:i32)
            n148 = call "Get PSU Field.vi"("error in (no error)"=w408, "Instrument.1820 in"=w409) -> ("error out"=w420:errorcluster, "PSU Field (T)"=w422:dbl, "Instrument.1820 in"=w421:refnum<class "Instrument.OxfordVRM.lvclass">)  [unwired: 7 in]
            n149 = call "FloatApprox.vi"("y"=w414, "x"=w422) -> ("x ~ y?"=w423:bool)  [unwired: 4 in]
            n150 = case shown="False" w423 {
              tunnel: [w428 w437] -> _
              tunnel: [w430 w436] -> w413
              tunnel: w421 -> [w433 w437]
              tunnel: w420 -> [w432 w436]
              tunnel: w414 -> [w435 _]
              tunnel: w415 -> [w434 _]
              tunnel: w407 -> [w427 _]
              frame False {
                n151 = call "Set Target.vi"("Axis"=w427, "error in (no error)"=w432, "Target Rate (T/min)"=w434, "Target Field (T)"=w435, "Instrument.VRM in"=w433) -> ("error out"=w431:errorcluster, "Instrument.VRM out"=w429:refnum<class "Instrument.OxfordVRM.lvclass">)  [unwired: 4 in, 1 out]
                n152 = call "Ramp to Set.vi"("Axis"=w427, "error in (no error)"=w431, "Instrument.VRM in"=w429) -> ("error out"=w430:errorcluster, "Instrument.VRM out"=w428:refnum<class "Instrument.OxfordVRM.lvclass">)  [unwired: 6 in, 1 out]
              }
              frame True {
                # "If PSU Field == Target, do nothing"
              }
            }
            n153 = Bundle By Name(cluster=w419, "Running Step"=w416) -> (w418:T6)
            n154 = call <vilib>:"Build State String with Arguments__JKI_lib_State_Machine.vi"("Arguments (\"\")"=w410, "State"="Sequence: Update Status") -> ("State with Arguments"=w411:string)  [unwired: 4 in]
            n155 = call <vilib>:"Add State(s) to Queue__jki_lib_state_machine.vi"("State(s) in Front (\"\")"=w411, "State(s) in (\"\")"=w426) -> ("States Out"=w425:string)  [unwired: 13 in]
          }
          frame "Sequence: Ramp PSU to Magnet" {
            # "#todo\ndelete??"
            # "#todo: add abort public method"
            # "#todo: make these separate states\n1. check B = Target?\n2. Turn on switch\n3. set PSU to target\n4. check hold OR psu = target\n5. set persist mode"
            n156 = Unbundle By Name(w454) -> ("Running Step"=w452:i32, "Self Reference"=w440:refnum<class "Instrument.OxfordVRM.lvclass">, "Axis"=w438:T5)  [unwired: 2 out]
            n157 = call "Get PSU Field.vi"("error in (no error)"=w439, "Instrument.1820 in"=w440) -> ("error out"=w444:errorcluster, "PSU Field (T)"=w445:dbl, "Instrument.1820 in"=w446:refnum<class "Instrument.OxfordVRM.lvclass">)  [unwired: 7 in]
            n158 = Increment(x=w452) -> (x+1=w451:i32)
            n159 = call "Get Field.vi"("error in (no error)"=w444, "Instrument.VRM in"=w446) -> ("error out"=w448:errorcluster, "Field (T)"=w447:dbl, "Instrument.VRM out"=w449:refnum<class "Instrument.OxfordVRM.lvclass">)  [unwired: 7 in]
            n160 = call "FloatApprox.vi"("y"=w445, "x"=w447) -> ("x ~ y?"=w455:bool)  [unwired: 4 in]
            n161 = case shown="False" w455 {
              tunnel: [w462 w469] -> _
              tunnel: [w464 w468] -> w450
              tunnel: w449 -> [w467 w469]
              tunnel: w448 -> [w466 w468]
              tunnel: w447 -> [w461 _]
              tunnel: w438 -> [w459 _]
              frame False {
                n162 = call "Set Target.vi"("Axis"=w459, "error in (no error)"=w466, "Target Rate (T/min)"=1.0, "Target Field (T)"=w461, "Instrument.VRM in"=w467) -> ("error out"=w465:errorcluster, "Instrument.VRM out"=w463:refnum<class "Instrument.OxfordVRM.lvclass">)  [unwired: 4 in, 1 out]
                n163 = call "Ramp to Set.vi"("Axis"=w459, "error in (no error)"=w465, "Instrument.VRM in"=w463) -> ("error out"=w464:errorcluster, "Instrument.VRM out"=w462:refnum<class "Instrument.OxfordVRM.lvclass">)  [unwired: 6 in, 1 out]
              }
              frame True {
                # "If PSU Field == Magnet, do nothing"
              }
            }
            n164 = Bundle By Name(cluster=w454, "Running Step"=w451) -> (w453:T6)
            n165 = call <vilib>:"Build State String with Arguments__JKI_lib_State_Machine.vi"("Arguments (\"\")"=w441, "State"="Sequence: Update Status") -> ("State with Arguments"=w442:string)  [unwired: 4 in]
            n166 = call <vilib>:"Add State(s) to Queue__jki_lib_state_machine.vi"("State(s) in Front (\"\")"=w442, "State(s) in (\"\")"=w458) -> ("States Out"=w457:string)  [unwired: 13 in]
          }
          frame "Sequence: Ramp PSU to Zero" {
            # "#todo: add abort public method"
            # "#todo: make these separate states\n1. check B = Target?\n2. Turn on switch\n3. set PSU to target\n4. check hold OR psu = target\n5. set persist mode"
            n167 = Unbundle By Name(w480) -> ("Running Step"=w478:i32, "Self Reference"=w473:refnum<class "Instrument.OxfordVRM.lvclass">, "Axis"=w470:T5)
            n168 = call "Ramp to Zero.vi"("Axis"=w470, "error in (no error)"=w472, "Instrument.VRM in"=w473) -> ("error out"=w471:errorcluster)  [unwired: 6 in, 2 out]
            n169 = Increment(x=w478) -> (x+1=w477:i32)
            n170 = Bundle By Name(cluster=w480, "Running Step"=w477) -> (w479:T6)
            n171 = call <vilib>:"Build State String with Arguments__JKI_lib_State_Machine.vi"("Arguments (\"\")"=w475, "State"="Sequence: Update Status") -> ("State with Arguments"=w474:string)  [unwired: 4 in]
            n172 = call <vilib>:"Add State(s) to Queue__jki_lib_state_machine.vi"("State(s) in Front (\"\")"=w474, "State(s) in (\"\")"=w483) -> ("States Out"=w482:string)  [unwired: 13 in]
          }
          frame "Sequence: Check Hold" {
            # "F = repeat this state. wait\nT = go to next state. don't wait"
            n173 = Unbundle By Name(w497) -> ("Running Step"=w499:i32, "Self Reference"=w493:refnum<class "Instrument.OxfordVRM.lvclass">, "Axis"=w485:T5)
            n174 = call "Get Status.vi"("Axis"=w485, "error in (no error)"=w484, "Instrument.VRM in"=w493) -> ("error out"=w487:errorcluster, "Status"=w501:T10)  [unwired: 5 in, 2 out]
            n175 = Unbundle By Name(w501) -> ("Holding"=w488:bool)
            n176 = Increment(x=w499) -> (x+1=w500:i32)
            n177 = Select(t=w500, s=w488, f=w499) -> (s? t:f=w498:i32)
            n178 = Select(t=u32 0, s=w488, f=u32 500 ("milliseconds to wait")) -> (s? t:f=w490:u32)
            n179 = Bundle By Name(cluster=w497, "Running Step"=w498) -> (w496:T6)
            n180 = call <userlib>:"Wait (ms)__ogtk.vi"("error in (no error)"=w487, "milliseconds to wait"=w490) -> ("error out"=w486:errorcluster)  [unwired: 8 in, 1 out]
            n181 = call <vilib>:"Build State String with Arguments__JKI_lib_State_Machine.vi"("Arguments (\"\")"=w494, "State"="Sequence: Update Status") -> ("State with Arguments"=w492:string)  [unwired: 4 in]
            n182 = call <vilib>:"Add State(s) to Queue__jki_lib_state_machine.vi"("State(s) in Front (\"\")"=w492, "State(s) in (\"\")"=w504) -> ("States Out"=w503:string)  [unwired: 13 in]
          }
          frame "Sequence: Check RTOS" {
            # "F = repeat this state. wait\nT = go to next state. don't wait"
            n183 = Unbundle By Name(w518) -> ("Running Step"=w520:i32, "Self Reference"=w514:refnum<class "Instrument.OxfordVRM.lvclass">, "Axis"=w505:T5)
            n184 = call "Get Status.vi"("Axis"=w505, "error in (no error)"=w506, "Instrument.VRM in"=w514) -> ("error out"=w508:errorcluster, "Status"=w522:T10)  [unwired: 5 in, 2 out]
            n185 = Unbundle By Name(w522) -> ("Ramp to Setpoint"=w509:bool)
            n186 = Increment(x=w520) -> (x+1=w521:i32)
            n187 = Select(t=w521, s=w509, f=w520) -> (s? t:f=w519:i32)
            n188 = Select(t=u32 0, s=w509, f=u32 500 ("milliseconds to wait")) -> (s? t:f=w511:u32)
            n189 = Bundle By Name(cluster=w518, "Running Step"=w519) -> (w517:T6)
            n190 = call <userlib>:"Wait (ms)__ogtk.vi"("error in (no error)"=w508, "milliseconds to wait"=w511) -> ("error out"=w507:errorcluster)  [unwired: 8 in, 1 out]
            n191 = call <vilib>:"Build State String with Arguments__JKI_lib_State_Machine.vi"("Arguments (\"\")"=w515, "State"="Sequence: Update Status") -> ("State with Arguments"=w513:string)  [unwired: 4 in]
            n192 = call <vilib>:"Add State(s) to Queue__jki_lib_state_machine.vi"("State(s) in Front (\"\")"=w513, "State(s) in (\"\")"=w525) -> ("States Out"=w524:string)  [unwired: 13 in]
          }
          frame "Sequence: Check RTOZ" {
            # "F = repeat this state. wait\nT = go to next state. don't wait"
            n193 = Unbundle By Name(w539) -> ("Running Step"=w541:i32, "Self Reference"=w535:refnum<class "Instrument.OxfordVRM.lvclass">, "Axis"=w526:T5)
            n194 = call "Get Status.vi"("Axis"=w526, "error in (no error)"=w527, "Instrument.VRM in"=w535) -> ("error out"=w529:errorcluster, "Status"=w543:T10)  [unwired: 5 in, 2 out]
            n195 = Unbundle By Name(w543) -> ("Ramp to Zero"=w530:bool)
            n196 = Increment(x=w541) -> (x+1=w542:i32)
            n197 = Select(t=w542, s=w530, f=w541) -> (s? t:f=w540:i32)
            n198 = Bundle By Name(cluster=w539, "Running Step"=w540) -> (w538:T6)
            n199 = Select(t=u32 0, s=w530, f=u32 500 ("milliseconds to wait")) -> (s? t:f=w532:u32)
            n200 = call <userlib>:"Wait (ms)__ogtk.vi"("error in (no error)"=w529, "milliseconds to wait"=w532) -> ("error out"=w528:errorcluster)  [unwired: 8 in, 1 out]
            n201 = call <vilib>:"Build State String with Arguments__JKI_lib_State_Machine.vi"("Arguments (\"\")"=w536, "State"="Sequence: Update Status") -> ("State with Arguments"=w534:string)  [unwired: 4 in]
            n202 = call <vilib>:"Add State(s) to Queue__jki_lib_state_machine.vi"("State(s) in Front (\"\")"=w534, "State(s) in (\"\")"=w546) -> ("States Out"=w545:string)  [unwired: 13 in]
          }
          frame "Sequence: Check PSU at Zero" {
            # "#todo\nnot needed???"
            # "F = repeat this state. wait\nT = go to next state. don't wait"
            n203 = Unbundle By Name(w564) -> ("Running Step"=w559:i32, "Self Reference"=w554:refnum<class "Instrument.OxfordVRM.lvclass">)
            n204 = call "Get PSU Field.vi"("error in (no error)"=w549, "Instrument.1820 in"=w554) -> ("error out"=w548:errorcluster, "PSU Field (T)"=w562:dbl)  [unwired: 7 in, 1 out]
            n205 = call "FloatApprox.vi"("y"=0.0, "x"=w562) -> ("x ~ y?"=w550:bool)  [unwired: 4 in]
            n206 = Increment(x=w559) -> (x+1=w560:i32)
            n207 = Select(t=w560, s=w550, f=w559) -> (s? t:f=w558:i32)
            n208 = Bundle By Name(cluster=w564, "Running Step"=w558) -> (w563:T6)
            n209 = Select(t=u32 0, s=w550, f=u32 500 ("milliseconds to wait")) -> (s? t:f=w552:u32)
            n210 = call <userlib>:"Wait (ms)__ogtk.vi"("error in (no error)"=w548, "milliseconds to wait"=w552) -> ("error out"=w547:errorcluster)  [unwired: 8 in, 1 out]
            n211 = call <vilib>:"Build State String with Arguments__JKI_lib_State_Machine.vi"("Arguments (\"\")"=w555, "State"="Sequence: Update Status") -> ("State with Arguments"=w556:string)  [unwired: 4 in]
            n212 = call <vilib>:"Add State(s) to Queue__jki_lib_state_machine.vi"("State(s) in Front (\"\")"=w556, "State(s) in (\"\")"=w567) -> ("States Out"=w566:string)  [unwired: 13 in]
          }
          frame "Sequence: Check Targets Match" {
            w571 = "" ("State")
            # "F = repeat this state. wait\nT = go to next state. don't wait"
            n213 = Unbundle By Name(w592) -> ("Running Step"=w589:i32, "Self Reference"=w581:refnum<class "Instrument.OxfordVRM.lvclass">, "Field (T)"=w577:dbl, "Field Rate (T/min)"=w575:dbl, "Axis"=w568:T5)
            n214 = call "Get Target.vi"("Axis"=w568, "error in (no error)"=w580, "Instrument.VRM in"=w581) -> ("error out"=w579:errorcluster, "Target Field Rate (T/min)"=w576:dbl, "Target Field (T)"=w578:dbl)  [unwired: 5 in, 1 out]
            n215 = call "FloatApprox.vi"("y"=w577, "x"=w578) -> ("x ~ y?"=w574:bool)  [unwired: 4 in]
            n216 = call "FloatApprox.vi"("y"=w575, "x"=w576) -> ("x ~ y?"=w573:bool)  [unwired: 4 in]
            n217 = Increment(x=w589) -> (x+1=w590:i32)
            n218 = And(x=w574, y=w573) -> (x .and. y?=w572:bool)
            n219 = Select(t=w590, s=w572, f=w589) -> (s? t:f=w588:i32)
            n220 = Select(t=u32 0, s=w572, f=u32 500 ("milliseconds to wait")) -> (s? t:f=w583:u32)
            n221 = Select(t=w571, s=w572, f=w571) -> (s? t:f=w570:string)
            n222 = call <userlib>:"Wait (ms)__ogtk.vi"("error in (no error)"=w579, "milliseconds to wait"=w583) -> ("error out"=w585:errorcluster)  [unwired: 8 in, 1 out]
            n223 = Bundle By Name(cluster=w592, "Running Step"=w588) -> (w591:T6)
            n224 = call <vilib>:"Build State String with Arguments__JKI_lib_State_Machine.vi"("Arguments (\"\")"=w570, "State"=w570) -> ()  [unwired: 4 in, 1 out]
            n225 = call <vilib>:"Build State String with Arguments__JKI_lib_State_Machine.vi"("Arguments (\"\")"=w586, "State"="Sequence: Update Status") -> ("State with Arguments"=w569:string)  [unwired: 4 in]
            n226 = call <vilib>:"Add State(s) to Queue__jki_lib_state_machine.vi"("State(s) in Front (\"\")"=w569, "State(s) in (\"\")"=w595) -> ("States Out"=w594:string)  [unwired: 13 in]
          }
        }
      }
    }
    frame Error {
    }
  }
  n227 = call-parent "Process.vi"("error in"=w7, "Instrument"=w6) -> ("error out"=w4:errorcluster, "Instrument out"=→"Instrument.Example out":refnum<class "Instrument.OxfordVRM.lvclass">)  [unwired: 8 in]
  n228 = Merge Errors(w4, w3) -> (→"error out":errorcluster)
